vi "AuMT8852B Test Delay.vi"(5 "Number of packets (0)":i32, 7 "Set/Get (Set)":enum16{"Set", "Get"}(ring), 8 "error in (no error)":errorcluster, 10 "Script (3)":i32=3, 11 "VISA session":refnum<visa-resource-name>) -> (0 "error out":errorcluster, 2 "error code":i32, 3 "VISA session out":refnum<visa-resource-name>, 4 "Number of packets out":i32)   [LabVIEW 2017]
doc: "Anritsu MT8852B Bluetooth Tester\n\nSets the number of packets to wait before changing test controls.\n\nINPUTS\nSet/Get - whether the value is being sent to or retrieved from the instrument.\nScript - test script (1-10) for which the delay is being set or queried. Scripts 1 and 2 are read-only.\nNumber of packets - (0 to 1000) how long to wait.\n\nOUTPUTS\nNumber of packets out - how long the instrument will wait."
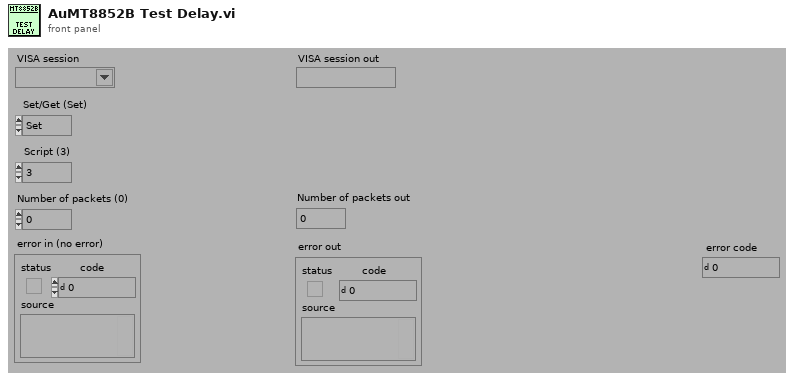
[diagram p1: front panel]
types:
  T1 = enum16{"Simulate", "Range check", "Cache", "Query instrument status"}
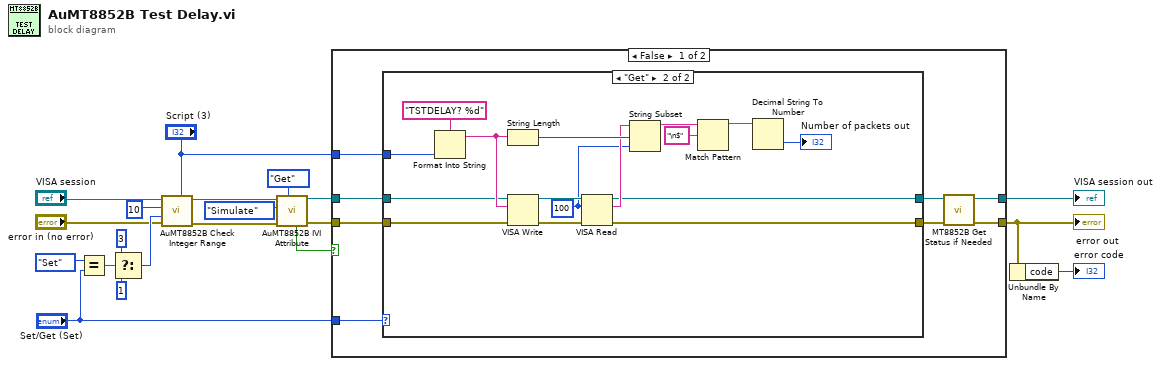
[diagram p0: block diagram]
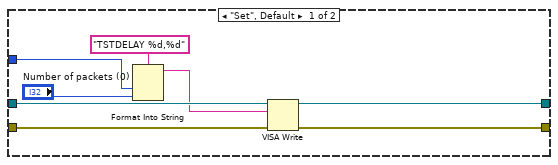
[diagram p2: hidden frame]
diagram:
  n1 = Equal?(x=enum16{"Set", "Get"}."Set" ("y"), y="Set/Get (Set)") -> (x = y?=w12:bool)
  n2 = Select(t=3, s=w12, f=1) -> (s? t:f=w9:i32)
  n3 = call <instrlib>:"AuMT8852B Check Integer Range.vi"("Value (0)"="Script (3)", "error in (no error)"="error in (no error)", "Lower limit (-1)"=w9, "Upper limit (1)"=10, "VISA session"="VISA session") -> ("error out"=w6:errorcluster, "VISA session out"=w7:refnum<visa-resource-name>)  [unwired: 5 in]
  n4 = call <instrlib>:"AuMT8852B IVI Attribute.vi"("Set/Get (Set)"=enum16{"Set", "Get"}."Get", "error in (no error)"=w6, "Flag (Simulate)"=T1."Simulate", "VISA session"=w7) -> ("error out"=w16:errorcluster, "VISA session out"=w17:refnum<visa-resource-name>, "Value out"=w15:bool)  [unwired: 5 in]
  n5 = case shown="False" w15 {
    tunnel: [w25 w53] -> w20
    tunnel: [w24 w54] -> w13
    tunnel: w17 -> [w28 w53]
    tunnel: w16 -> [w27 w54]
    tunnel: "Script (3)" -> [w22 _]
    tunnel: "Set/Get (Set)" -> [w21 _]
    frame False {
      n6 = case shown="\"Get\"" w21 {
        tunnel: w28 -> [w36 w44]
        tunnel: w27 -> [w35 w43]
        tunnel: [w34 w42] -> w26
        tunnel: [w33 w41] -> w23
        tunnel: w22 -> [w29 w40]
        frame "Set", Default {
          n7 = Format Into String(format string="TSTDELAY %d,%d" ("Format String"), w29, "Number of packets (0)") -> (resulting string=w31:string)  [unwired: 2 in, 1 out]
          n8 = VISA Write(VISA resource name=w36, write buffer=w31, error in (no error)=w35) -> (VISA resource name out=w34:refnum<visa-resource-name>, error out=w33:errorcluster)  [unwired: 1 out]
        }
        frame "Get" {
          w37 = u32 100 ("byte count (0)")
          n9 = Format Into String(format string="TSTDELAY? %d" ("Format String"), w40) -> (resulting string=w48:string)  [unwired: 2 in, 1 out]
          n10 = String Length(string=w48) -> (length=w47:i32)
          n11 = VISA Write(VISA resource name=w44, write buffer=w48, error in (no error)=w43) -> (VISA resource name out=w52:refnum<visa-resource-name>, error out=w51:errorcluster)  [unwired: 1 out]
          n12 = VISA Read(VISA resource name=w52, byte count=w37, error in (no error)=w51) -> (VISA resource name out=w42:refnum<visa-resource-name>, read buffer=w45:string, error out=w41:errorcluster)  [unwired: 1 out]
          n13 = String Subset(string=w45, offset (0)=w47, length (rest)=w37) -> (substring=w46:string)
          n14 = Match Pattern(string=w46, regular expression="\n$") -> (before substring=w39:string)  [unwired: 1 in, 3 out]
          n15 = Decimal String To Number(string=w39) -> (number=→"Number of packets out":i32)  [unwired: 2 in, 1 out]
        }
      }
      n16 = call <instrlib>:"MT8852B Get Status if Needed.vi"("error in (no error)"=w23, "VISA session"=w26) -> ("error out"=w24:errorcluster, "VISA session out"=w25:refnum<visa-resource-name>)  [unwired: 8 in]
    }
    frame True {
    }
  }
  "VISA session out" <- w20
  "error out" <- w13
  n17 = Unbundle By Name(w13) -> ("code"=→"error code":i32)
